vi "Select Format File.vi"(8 "error in (no error)":errorcluster, 10 "Formato":enum16{"txt", "csv"}(ring), 11 "F Generator in":refnum<class "F Generator.lvclass">) -> (0 "error out":errorcluster, 3 "F Generator out":refnum<class "F Generator.lvclass">)   [LabVIEW 2020, in "F Generator.lvlib" / "F Generator.lvclass"]
uses:
  F Generator.lvclass
  C:/Program Files/National Instruments/LabVIEW 2020/vi.lib/ActorFramework/Actor/Actor.lvclass
  F Generator.lvclass/F Generator.ctl
  Text Actor/Text Actor/Text Actor.lvclass
  CSV Actor/CSV Actor/CSV Actor.lvclass
  C:/Users/deLili/Desktop/UDLSB IET/701/Instrumentacion Virtual/Fork/AF-CML-TAREA/AF-CML-Tarea/Text Actor/Text Actor/Text Actor.lvclass
  <vilib>/ActorFramework/Message Enqueuer/Message Enqueuer.lvclass/Message Enqueuer.ctl
  <vilib>/ActorFramework/Message Enqueuer/Enqueue.vi
  <vilib>/ActorFramework/Stop Msg/Stop Msg.lvclass
  C:/Program Files/National Instruments/LabVIEW 2020/vi.lib/ActorFramework/Message/Message.lvclass
  <vilib>/ActorFramework/Message Priority Queue/Priority Enqueue.vi
  <vilib>/ActorFramework/Actor/Actor.lvclass
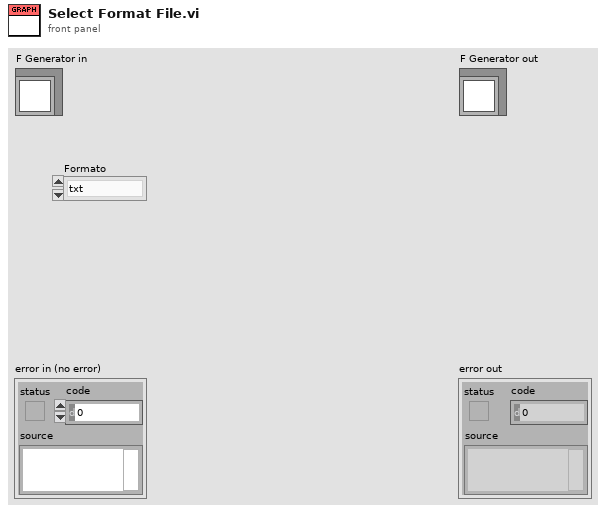
[diagram p1: front panel]
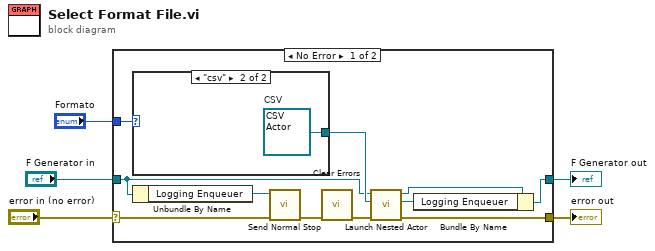
[diagram p0: block diagram]
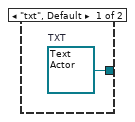
[diagram p2: hidden frame]
diagram:
  n1 = case shown="No Error" "error in (no error)" {
    selector: "error in (no error)" -> [w15 w20]
    tunnel: [w12 w20] -> w4
    tunnel: [w8 w19] -> w2
    tunnel: "F Generator in" -> [w10 w19]
    tunnel: "Formato" -> [w16 _]
    frame No Error {
      n2 = case shown="\"csv\"" w16 {
        tunnel: [w17 w18] -> w11
        frame "txt", Default {
          w17 = refnum<class "Text Actor.lvclass"> refnum  # TXT
        }
        frame "csv" {
          w18 = refnum<class "CSV Actor.lvclass"> refnum  # CSV
        }
      }
      n3 = Unbundle By Name(w10) -> ("Logging Enqueuer"=w6:refnum<class "Message Enqueuer.lvclass">)
      n4 = call <vilib>:"Send Normal Stop.vi"("error in (no error)"=w15, "Message Enqueuer"=w6) -> ("error out"=w14:errorcluster)  [unwired: 9 in]
      n5 = call <vilib>:"Clear Errors.vi"("error in (no error)"=w14) -> ("error out"=w13:errorcluster)  [unwired: 5 in, 1 out]
      n6 = call <vilib>:"Launch Nested Actor.vi"("error in (no error)"=w13, "Nested Actor"=w11, "Caller Actor in"=w10) -> ("error out"=w12:errorcluster, "Nested Actor's Enqueuer"=w7:refnum<class "Message Enqueuer.lvclass">, "Caller Actor out"=w9:refnum<class "F Generator.lvclass">)  [unwired: 6 in]
      n7 = Bundle By Name(cluster=w9, "Logging Enqueuer"=w7) -> (w8:refnum<class "F Generator.lvclass">)
    }
    frame Error {
    }
  }
  "error out" <- w4
  "F Generator out" <- w2
